vi "exemple_mesureForce.vi"() -> ()   [LabVIEW 2010]
panel:
  out "data":dbl
  out "Waveform Chart":dynamicdata(graph)
  in  "stop":bool
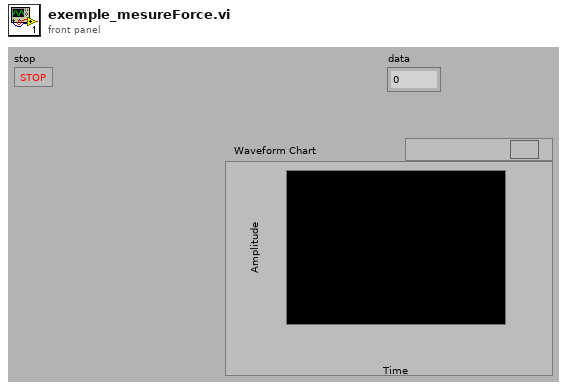
[diagram p1: front panel]
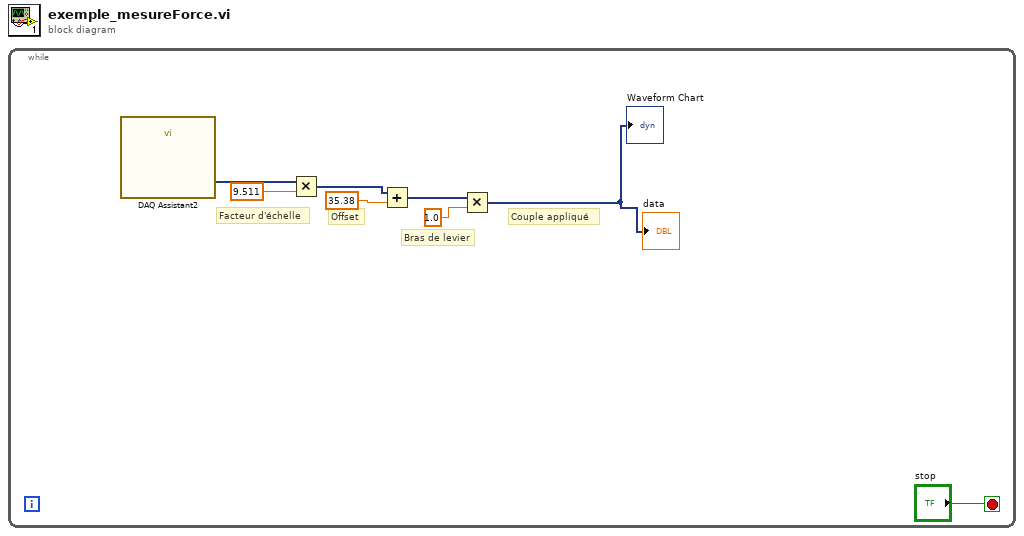
[diagram p0: block diagram]
diagram:
  n1 = while {
    stop <- "stop" stop-if-true
    # "Bras de levier"
    # "Couple appliqué"
    # "Offset"
    # "Facteur d'échelle"
    n2 = call "DAQ Assistant2"() -> ("data"=w7:dynamicdata)  [unwired: 17 in, 2 out]
    n3 = Multiply(x=w7, y=9.511) -> (x*y=w5:dynamicdata)
    n4 = Add(x=w5, y=35.38) -> (x+y=w3:dynamicdata)
    n5 = Multiply(x=w3, y=1.0) -> (x*y=→"Waveform Chart" →"data":dynamicdata)
  }
